vi "Unknown Messages.vi"(8 "error in (no error)":errorcluster, 10 "Message":string, 11 "Process In":refnum<class "Process.lvclass">) -> (0 "error out":errorcluster, 3 "Process Out":refnum<class "Process.lvclass">)   [LabVIEW 2020, in "Process.lvclass"]
uses:
  Process.lvclass
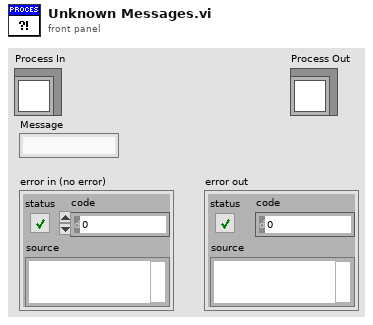
[diagram p1: front panel]
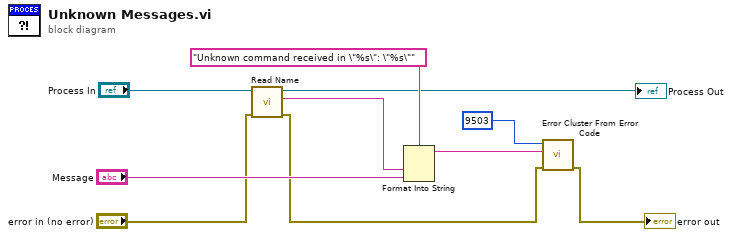
[diagram p0: block diagram]
diagram:
  n1 = call-dynamic "Read Name.vi"("error in (no error)"="error in (no error)", "Process In"="Process In") -> ("error out"=w2:errorcluster, "Qualified Name"=w4:string, "Process Out"=→"Process Out":refnum<class "Process.lvclass">)  [unwired: 6 in, 1 out]
  n2 = Format Into String(format string="Unknown command received in \"%s\": \"%s\"", w4, "Message") -> (resulting string=w10:string)  [unwired: 2 in, 1 out]
  n3 = call <vilib>:"Error Cluster From Error Code.vi"("error in (no error)"=w2, "error message (\"\")"=w10, "error code (0)"=9503) -> ("error out"=→"error out":errorcluster)  [unwired: 6 in]
